vi "Reset Output Protection.vi"(8 "error in (no error)":errorcluster, 11 "VISA resource name":refnum<visa-resource-name>) -> (0 "error out":errorcluster, 3 "VISA resource name out":refnum<visa-resource-name>)   [LabVIEW 2013]
doc: "This VI resets the power supply's output protection after an over-voltage.\n\nAn over-voltage condition occurs when the output voltage is equal to or greater than the OVP value and that OVP is enabled. \n\nWhen an over-voltage condition occurs, the output protection of the power supply disables the output. Once the output protection is reset, the power supply resumes generating a power signal.\n\nYou use the hpe364xa Query Output State VI to determine if the power supply is in an output-protection state."
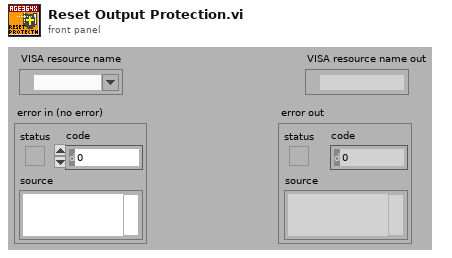
[diagram p1: front panel]
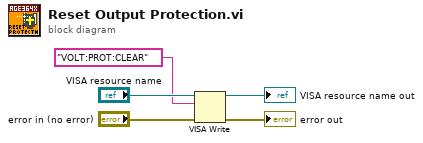
[diagram p0: block diagram]
diagram:
  n1 = VISA Write(VISA resource name="VISA resource name", write buffer="VOLT:PROT:CLEAR", error in (no error)="error in (no error)") -> (VISA resource name out=→"VISA resource name out":refnum<visa-resource-name>, error out=→"error out":errorcluster)  [unwired: 1 out]
